vi "replace text in Word doc.vi"(8 "Error In (no error)":errorcluster) -> (0 "Error Out":errorcluster)   [LabVIEW 2015, in "AguaClara Library.lvlib"]
doc: "This VI will prompt the user for a PowerPoint slide show presentation *.pps file and then launch PowerPoint. The slide show will be run in a full screen."
uses:
  AguaClara Library.lvlib
panel:
  in  "Path":path=path "C:/Documents and Settings/mw24/Desktop/DesignReport2.docx"
  out "Update":i32
  out "result string":string
  in  "Replacewith":string
  in  "Find":string
  in  "Word._Application 2":refnum<k7>
  # "This program now searches a word documetn and replaces all instances of the FInd text. It then saves the file as a pdf and closes the original file without changes."
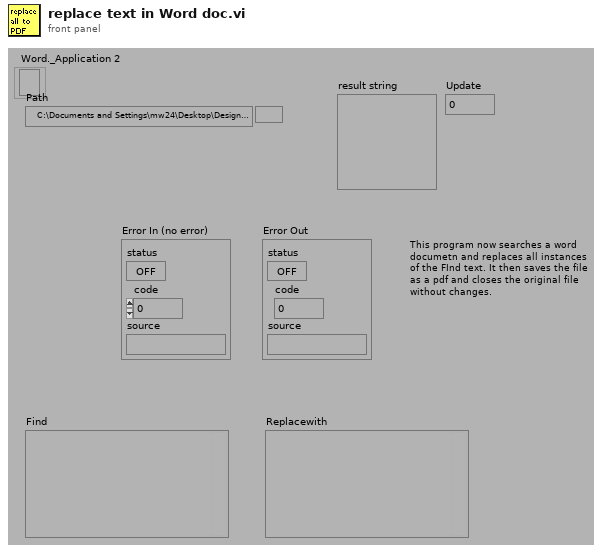
[diagram p1: front panel]
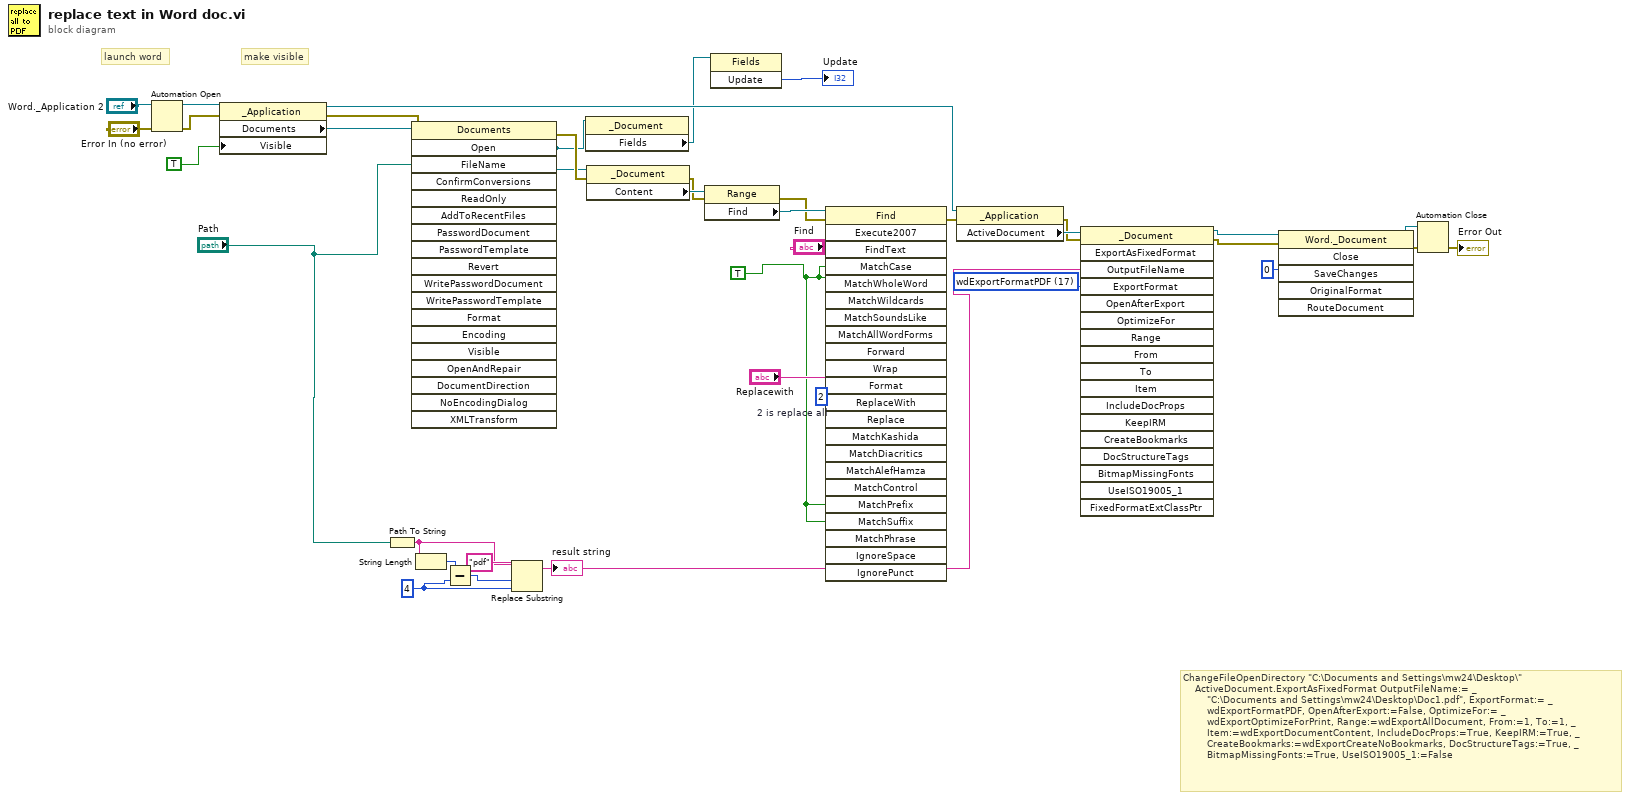
[diagram p0: block diagram]
diagram:
  w1 = TRUE ("Visible")
  w14 = 4 ("length (len. of substring)")
  w19 = 17 items=["wdExportFormatPDF"=17, "wdExportFormatXPS"=18] ("ExportFormat")
  w23 = 2  # 2 is replace all
  # "ChangeFileOpenDirectory \"C:\\Documents and Settings\\mw24\\Desktop\\\"\n    ActiveDocument.ExportAsFixedFormat OutputFileName:= _\n        \"C:\\Documents and Settings\\mw24\\Desktop\\Doc1.pdf\", ExportFormat:= _\n        wdExportFormatPDF, OpenAfterExport:=False, OptimizeFor:= _\n        wdExportOptimizeForPrint, Range:=wdExportAllDocument, From:=1, To:=1, _\n        Item:=wdExportDocumentContent, IncludeDocProps:=True, KeepIRM:=True, _\n        CreateBookmarks:=wdExportCreateNoBookmarks, DocStructureTags:=True, _\n        BitmapMissingFonts:=True, UseISO19005_1:=False"
  # "make visible"
  # "launch word"
  n1 = Automation Open(error in (no error)="Error In (no error)", Automation Refnum="Word._Application 2") -> (Automation Refnum=w2:refnum<k7>, error out=w35:errorcluster)  [unwired: 2 in]
  n2 = property class="_Application"(reference=w2, error in=w35, "Visible"=TRUE) -> (reference out=w22:refnum<k7>, error out=w32:errorcluster, "Documents"=w33:refnum<k7>)
  n3 = Path To String(path="Path") -> (string=w16:string)
  n4 = invoke class="Documents" method="Open"(reference=w33, error in=w32, "FileName"="Path") -> (error out=w31:errorcluster, "Open"=w5:refnum<k7>)  [unwired: 16 in, 17 out]
  n5 = String Length(string=w16) -> (length=w15:i32)
  n6 = Subtract(x=w15, y=w14) -> (x-y=w13:i32)
  n7 = Replace Substring(2:w14, 3:w13, 4:"pdf" ("substring (\"\")"), 5:w16) -> (1:w12:string)  [unwired: 1 out]
  "result string" <- w12
  n8 = property class="_Document"(reference=w5) -> ("Fields"=w4:refnum<k7>)  [unwired: 1 in, 2 out]
  n9 = property class="_Document"(reference=w5, error in=w31) -> (error out=w6:errorcluster, "Content"=w7:refnum<k7>)  [unwired: 1 out]
  n10 = property class="Range"(reference=w7, error in=w6) -> (error out=w25:errorcluster, "Find"=w26:refnum<k7>)  [unwired: 1 out]
  n11 = invoke class="Fields" method="Update"(reference=w4) -> ("Update"=→"Update":i32)  [unwired: 2 in, 2 out]
  n12 = invoke class="Find" method="Execute2007"(reference=w26, error in=w25, "FindText"="Find", "MatchCase"=w1, "MatchWholeWord"=w1, "ReplaceWith"="Replacewith", "Replace"=w23, "MatchPrefix"=w1, "MatchSuffix"=w1) -> (error out=w9:errorcluster)  [unwired: 14 in, 22 out]
  n13 = property class="_Application"(reference=w22, error in=w9) -> (error out=w20:errorcluster, "ActiveDocument"=w21:refnum<k7>)  [unwired: 1 out]
  n14 = invoke class="_Document" method="ExportAsFixedFormat"(reference=w21, error in=w20, "OutputFileName"=w12, "ExportFormat"=w19) -> (reference out=w11:refnum<k7>, error out=w10:errorcluster)  [unwired: 14 in, 16 out]
  n15 = invoke class="Word._Document" method="Close"(reference=w11, error in=w10, "SaveChanges"=0) -> (reference out=w29:refnum<k7>, error out=w30:errorcluster)  [unwired: 3 in, 4 out]
  n16 = Automation Close(3:w30, 5:w29) -> (0:→"Error Out":errorcluster)
